vi "Increment Iteration.vi"(8 "error in (no error)":errorcluster, 11 "Transfer Group in":refnum<class "Transfer Group.lvclass">) -> (0 "error out":errorcluster, 3 "Transfer Group out":refnum<class "Transfer Group.lvclass">)   [LabVIEW 2017, in "DSF Core.lvlib" / "Transfer Group.lvclass"]
uses:
  Transfer Group.lvclass
  Transfer Group.lvclass/Transfer Group.ctl
  Timing/Timing.lvclass
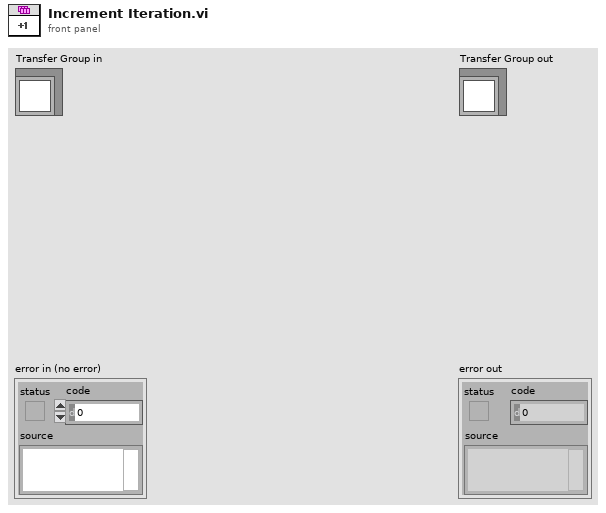
[diagram p1: front panel]
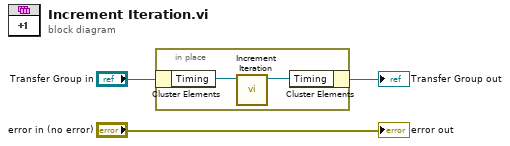
[diagram p0: block diagram]
diagram:
  n1 = in-place {
    n2 = in-place-cluster #1("Transfer Group in") -> ("Timing"=w5:refnum<class "Timing.lvclass">)
    n3 = call "Increment Iteration.vi"("Timing in"=w5) -> ("Timing out"=w4:refnum<class "Timing.lvclass">)  [unwired: 10 in]
    n4 = in-place-cluster #1("Timing"=w4) -> (→"Transfer Group out":refnum<class "Transfer Group.lvclass">)
  }
  "error out" <- "error in (no error)"
